vi "COM Port Handshake.vi"(8 "error in (no error)":errorcluster, 11 "VISA Refnum in":refnum<visa-resource-name>) -> (0 "error out":errorcluster, 2 "OptiTrack Connected?":bool, 3 "VISA Refnum out":refnum<visa-resource-name>)   [LabVIEW 2017]
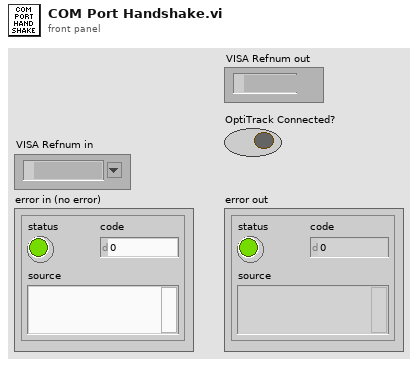
[diagram p1: front panel]
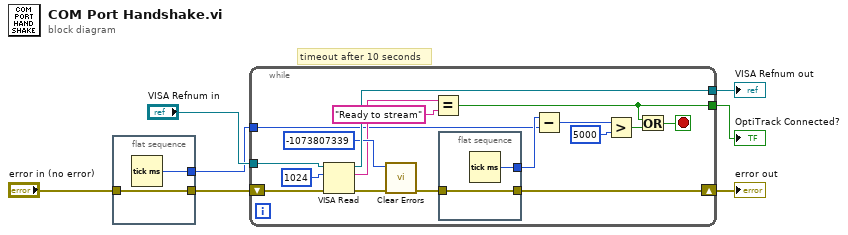
[diagram p0: block diagram]
diagram:
  # "timeout after 10 seconds"
  n1 = flat-sequence {
    tunnel: "error in (no error)" -> [w9]
    tunnel: [w9] -> w2
    tunnel: [w8] -> w1
    frame #0 {
      n2 = Tick Count (ms)() -> (millisecond timer value=w8:u32)
    }
  }
  n3 = while {
    shift-right: [w15] -> w5
    shift-left: w2 -> [w26]
    tunnel: "VISA Refnum in" -> [w25]
    tunnel: [w24] -> w4
    tunnel: [w18] -> w6
    tunnel: w1 -> [w13]
    stop <- w22 stop-if-true
    n4 = VISA Read(VISA resource name=w25, byte count=u32 1024, error in (no error)=w26) -> (VISA resource name out=w24:refnum<visa-resource-name>, read buffer=w17:string, error out=w21:errorcluster)  [unwired: 1 out]
    n5 = call <vilib>:"Clear Errors.vi"("error in (no error)"=w21, "specific error code to clear (0: all)"=-1073807339) -> ("error out"=w16:errorcluster)  [unwired: 4 in, 1 out]
    n6 = Equal?(x=w17, y="Ready to stream") -> (x = y?=w18:bool)
    n7 = flat-sequence {
      tunnel: w16 -> [w28]
      tunnel: [w28] -> w15
      tunnel: [w27] -> w14
      frame #0 {
        n8 = Tick Count (ms)() -> (millisecond timer value=w27:u32)
      }
    }
    n9 = Subtract(x=w14, y=w13) -> (x-y=w12:u32)
    n10 = Greater?(x=w12, y=u32 5000) -> (0:w10:bool)
    n11 = Or(x=w18, y=w10) -> (x .or. y?=w22:bool)
  }
  "OptiTrack Connected?" <- w6
  "error out" <- w5
  "VISA Refnum out" <- w4
